vi "get_num_ROIs.vi"(8 "error in (no error)":errorcluster, 11 "Hamamatsu_C9100-13 in":refnum<class "Hamamatsu_C9100-13.lvclass">) -> (0 "error out":errorcluster, 1 "shots per measurement":i32, 2 "number of ROI":i32, 3 "Hamamatsu_C9100-13 out":refnum<class "Hamamatsu_C9100-13.lvclass">)   [LabVIEW 2013, in "Hamamatsu_C9100-13.lvclass"]
uses:
  Hamamatsu_C9100-13.lvclass
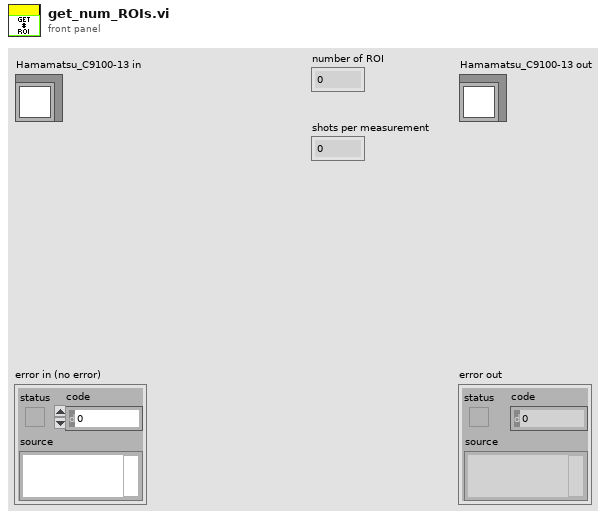
[diagram p1: front panel]
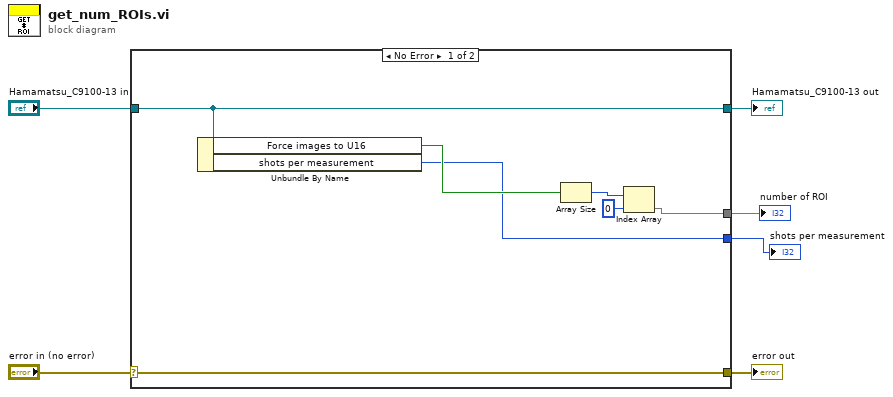
[diagram p0: block diagram]
diagram:
  n1 = case shown="No Error" "error in (no error)" {
    selector: "error in (no error)" -> [w13 w15]
    tunnel: [w13 w15] -> w5
    tunnel: [w12 w14] -> w3
    tunnel: "Hamamatsu_C9100-13 in" -> [w12 w14]
    tunnel: [w8 _] -> w2
    tunnel: [w7 _] -> w1
    frame No Error {
      n2 = Unbundle By Name(w12) -> ("Force images to U16"=w11:bool, "shots per measurement"=w7:i32)
      n3 = Array Size(array=w11) -> (size(s)=w10:i32)
      n4 = Index Array(array=w10, index=0) -> (element=w8)
    }
    frame Error {
    }
  }
  "error out" <- w5
  "Hamamatsu_C9100-13 out" <- w3
  "number of ROI" <- w2
  "shots per measurement" <- w1
